vi "Variant to JSON Text (inline TEST).vi"(5 "enable LabVIEW extensions? (T)":bool=TRUE, 6 "Pretty Print?":bool, 8 "error in (no error)":errorcluster, 10 "Variant":variant) -> (0 "error out":errorcluster, 3 "<JSON>":string)   [LabVIEW 2013, in "JSONtext.lvlib"]
doc: "Converts a LabVIEW datatype (<b>Variant</b>) into a JSON value. Clusters are converted to JSON Objects, or to an Array if the first cluster element is unnamed."
uses:
  JSONtext.lvlib
  support/Infinity&NaN.ctl
  <vilib>/Utility/VariantDataType/RefnumType.ctl
  <vilib>/Utility/VariantDataType/VariantType.lvlib
  support/JSONtext support.lvlib
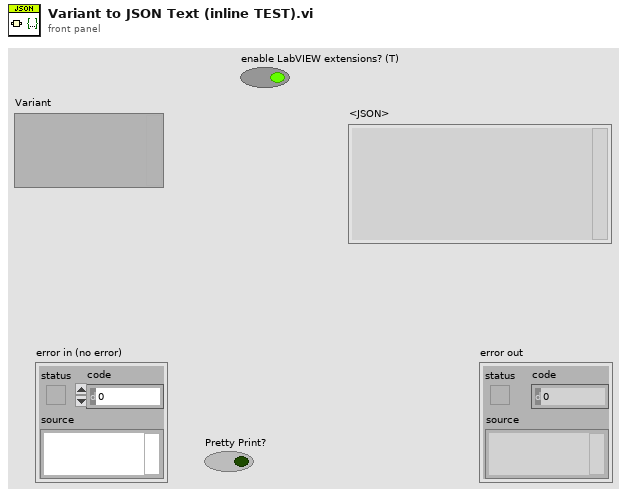
[diagram p1: front panel]
types:
  T1 = typedef "JSONtext support.lvlib/Infinity&NaN.ctl" = enum16{"Default (null)", "Extended", "LabVIEW extensions"}
  T2 = typedef "VariantType.lvlib/Type.ctl" = enum8{"Invalid Type", "Void", "I8", "I16", "I32", "I64", "U8", "U16", "U32", "U64", "Single Float", "Double Float", "Extended Float", "Single Complex", "Double Complex", "Extended Complex", "Enum U8", "Enum U16", "Enum U32", "Enum U64", "Single Float With Unit", "Double Float With Unit", "Extended Float With Unit", "Single Complex with Unit", "Double Complex with Unit", "Extended Complex with Unit", "Boolean", "String", "Path", "Picture", "Tag", "Array", "Cluster", "Variant", "LV Variant", "Waveform", "Timestamp", "Digital Waveform", "Digital Data", "ExpressData", "Refnum", "External Data", "VI", "Poly VI", "LabVIEW Class Instance", "Fixed Point"}
  T3 = cluster{"<JSON>attributes":string, "t0":timestamp, "dt":dbl, "Y":dbl[]}
  T4 = typedef "VariantType.lvlib/RefnumType.ctl" = enum16{"NotARefnum", "UnknownRefnum", "Generic", "Datalog", "ByteStream", "Device", "Occurence", "TCPNetConnection", "Auto", "Menu", "Imaq", "Hardware", "DataSocket", "Visa", "IVI", "UDPNetConnection", "Notifier", "Queue", "Irda", "EventReg", "DotNet", "UserEvent", "Callback", "UNUSED_EMPTY_POSITION", "BlueToothNetConnection", "LVObjApp", "LVObjVI", "LVObjUnknown", "GenericClass", "UserDefinedRefnumTag", "DataValue", "RT FIFO", "TDMS File"}
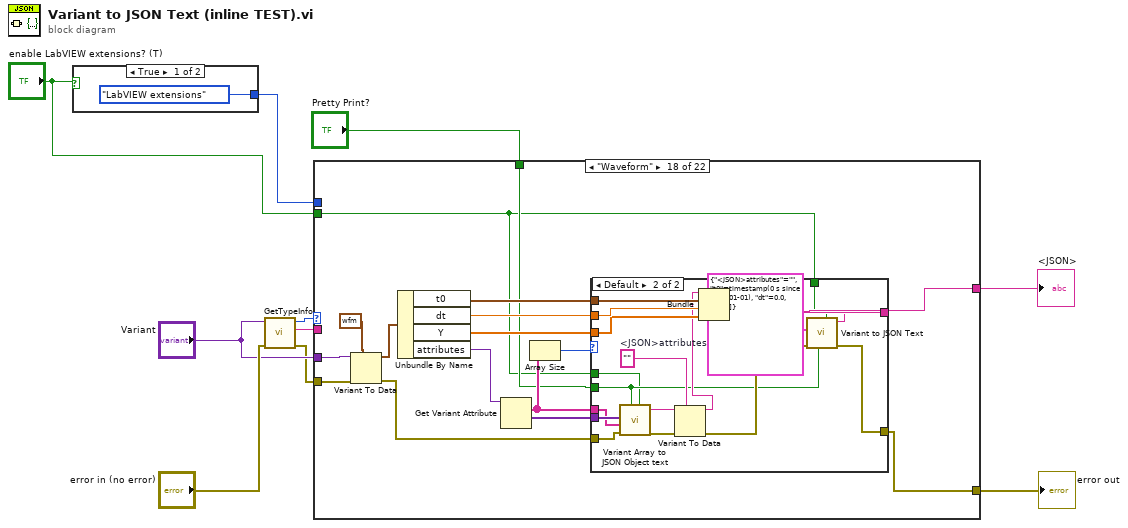
[diagram p0: block diagram]
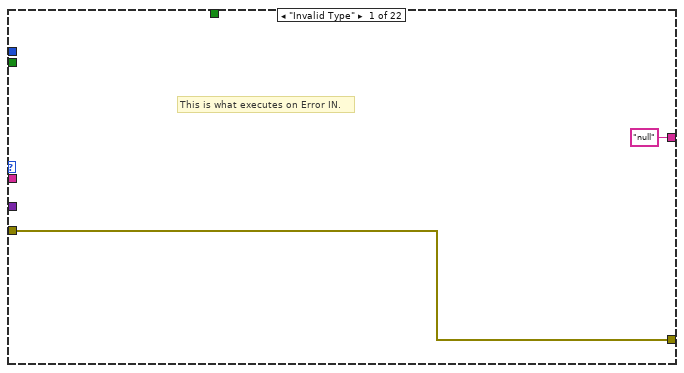
[diagram p2: hidden frame]
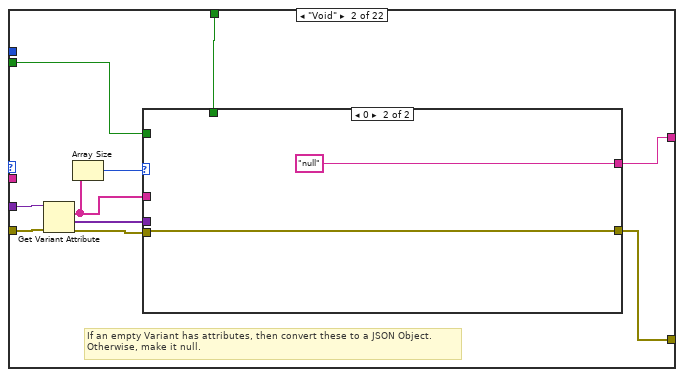
[diagram p3: hidden frame]
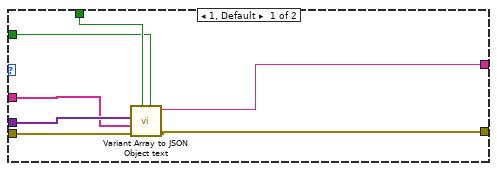
[diagram p4: hidden frame]
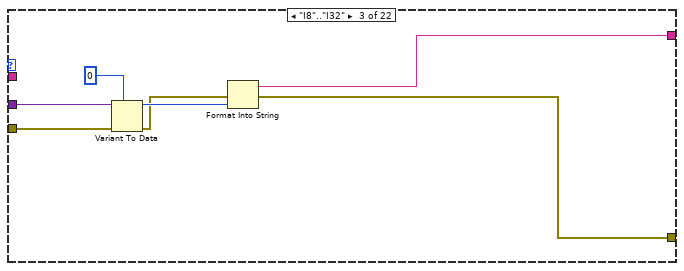
[diagram p5: hidden frame]
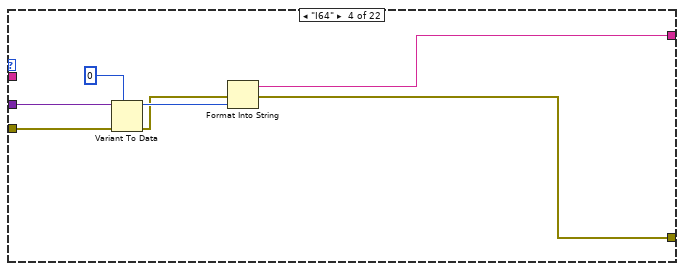
[diagram p6: hidden frame]
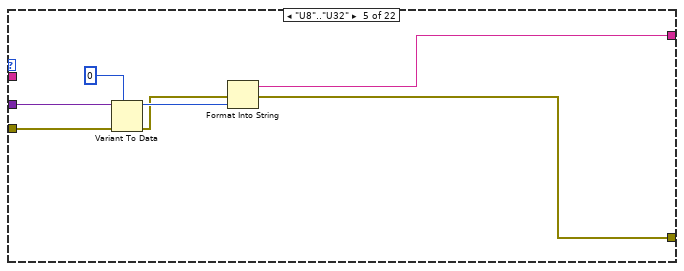
[diagram p7: hidden frame]
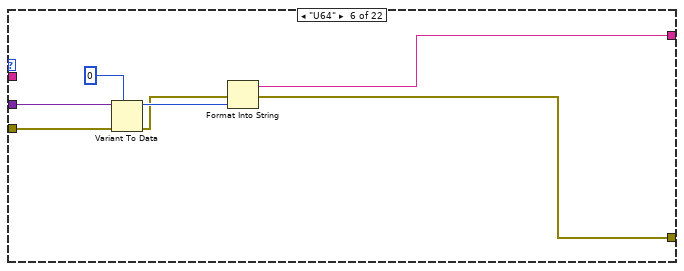
[diagram p8: hidden frame]
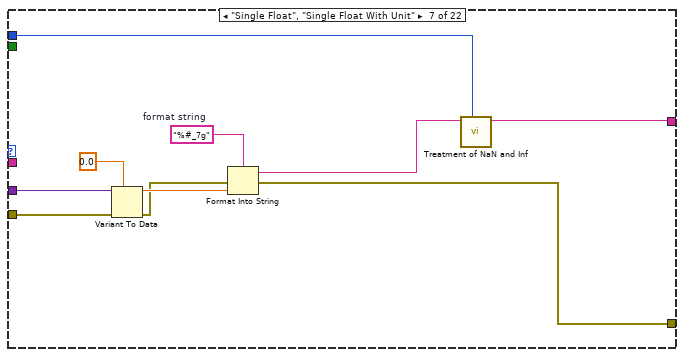
[diagram p9: hidden frame]
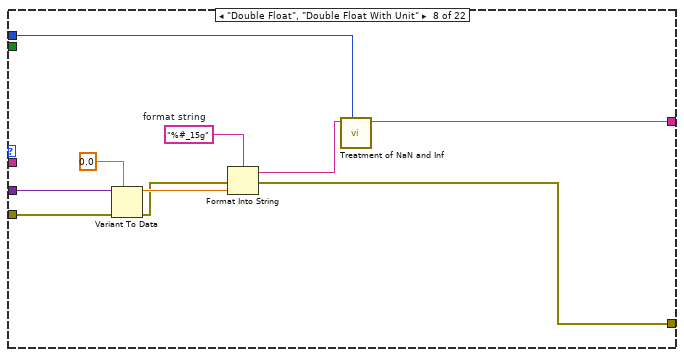
[diagram p10: hidden frame]
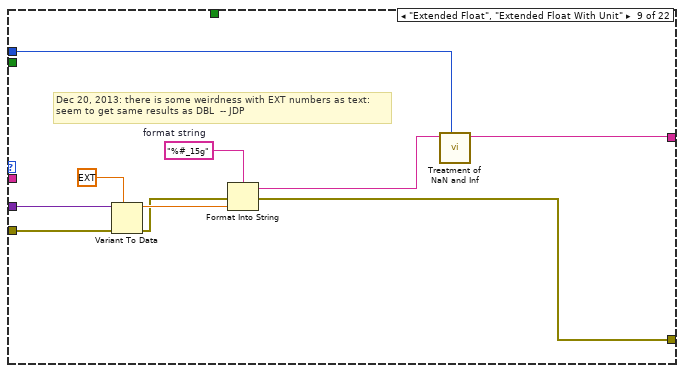
[diagram p11: hidden frame]
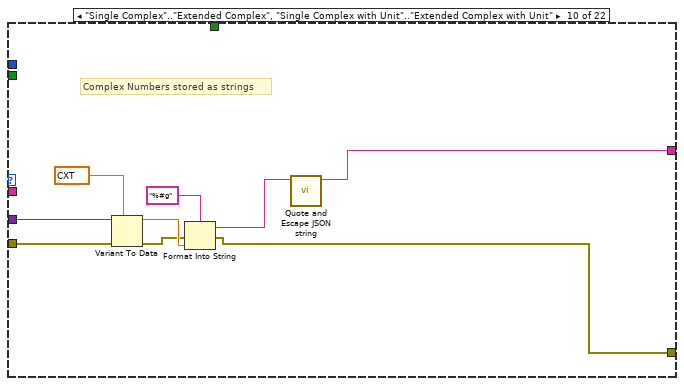
[diagram p12: hidden frame]
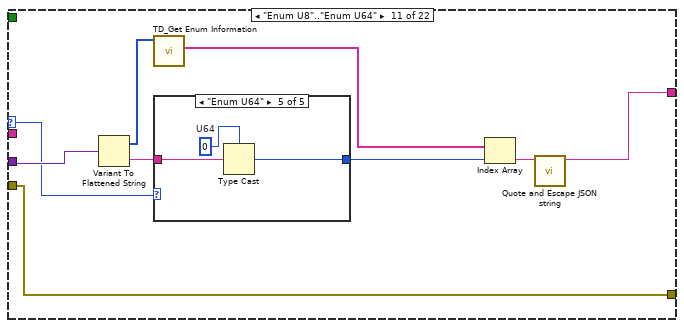
[diagram p13: hidden frame]
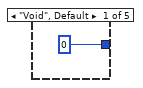
[diagram p14: hidden frame]
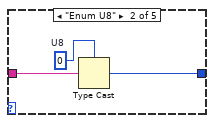
[diagram p15: hidden frame]
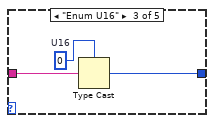
[diagram p16: hidden frame]
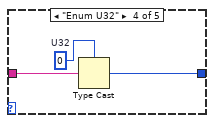
[diagram p17: hidden frame]
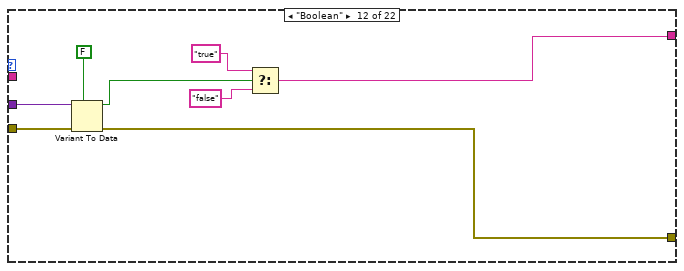
[diagram p18: hidden frame]
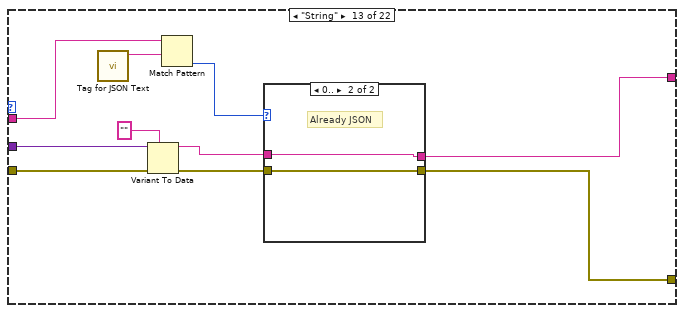
[diagram p19: hidden frame]
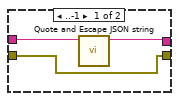
[diagram p20: hidden frame]
diagram:
  n1 = case shown="True" "enable LabVIEW extensions? (T)" {
    tunnel: [Infinity&NaN."LabVIEW extensions" ("Treatment of Infinity/NaN") Infinity&NaN."Default (null)" ("Treatment of Infinity/NaN")] -> w5
    frame True {
    }
    frame False {
    }
  }
  n2 = call <vilib>:"GetTypeInfo.vi"("error in (no error)"="error in (no error)", "Variant"="Variant") -> ("error out"=w3:errorcluster, "Name"=w1:string, "Type Enum"=w2:T2)  [unwired: 5 in, 2 out]
  n3 = case shown="\"Waveform\"" w2 {
    selector: w2 -> [_ _ _ _ _ _ _ _ _ _ w104 _ _ _ _ _ _ _ _ _ _ _]
    tunnel: "Variant" -> [_ w23 w40 w47 w54 w61 w71 w81 w91 w100 w105 w130 w140 w152 w163 w516 w533 w553 w588 w593 w619 w623]
    tunnel: [w13 w24 w34 w41 w48 w55 w66 w76 w86 w92 w101 w123 w136 w146 w164 w511 w537 w540 w580 w591 w612 w620] -> w9
    tunnel: w3 -> [w13 w18 w38 w45 w52 w59 w69 w79 w89 w99 w101 w128 w135 w150 w162 w514 w532 w552 w586 w592 w618 w620]
    tunnel: w1 -> [_ _ _ _ _ _ _ _ _ _ _ _ w133 _ w154 _ _ _ _ _ _ _]
    tunnel: w5 -> [_ _ _ _ _ _ w62 w72 w82 _ _ _ _ _ _ _ _ _ _ _ _ _]
    tunnel: ["null" ("<JSON>") w17 w36 w43 w50 w57 w63 w73 w83 w93 w102 w124 w131 w147 w156 w512 w529 w542 w581 w590 w615 w621] -> w7
    tunnel: "Pretty Print?" -> [_ w16 _ _ _ _ _ _ _ _ _ _ _ _ w157 w510 w531 w539 _ _ _ _]
    tunnel: "enable LabVIEW extensions? (T)" -> [_ w15 _ _ _ _ _ _ _ _ _ _ _ _ w155 w506 w530 w538 _ _ _ _]
    frame "Invalid Type" {
      # "This is what executes on Error IN."
    }
    frame "Void" {
      # "If an empty Variant has attributes, then convert these to a JSON Object.\nOtherwise, make it null."
      n4 = Get Variant Attribute(Variant=w23, error in=w18) -> (names=w21:string[], values=w20:variant[], error out=w19:errorcluster)  [unwired: 2 in, 1 out]
      n5 = Array Size(array=w21) -> (size(s)=w22:i32)
      n6 = case shown="0" w22 {
        tunnel: [w28 w32] -> w24
        tunnel: w21 -> [w30 _]
        tunnel: w20 -> [w31 _]
        tunnel: w19 -> [w29 w32]
        tunnel: [w27 "null"] -> w17
        tunnel: w16 -> [w26 _]
        tunnel: w15 -> [w25 _]
        frame 1, Default {
          n7 = call "Variant Array to JSON Object text.vi"("enable LabVIEW extensions? (T)"=w25, "Pretty Print?"=w26, "error in (no error)"=w29, "Names"=w30, "Array"=w31) -> ("error out"=w28:errorcluster, "<JSON>Object Text"=w27:string)  [unwired: 5 in]
        }
        frame 0 {
        }
      }
    }
    frame "I8".."I32" {
      n8 = Variant To Data(error in=w38, type=0, Variant=w40) -> (data=w37:i32, error out=w35:errorcluster)
      n9 = Format Into String(error in=w35, w37) -> (resulting string=w36:string, error out=w34:errorcluster)  [unwired: 2 in]
    }
    frame "I64" {
      n10 = Variant To Data(error in=w45, type=i64 0, Variant=w47) -> (data=w44:i64, error out=w42:errorcluster)
      n11 = Format Into String(error in=w42, w44) -> (resulting string=w43:string, error out=w41:errorcluster)  [unwired: 2 in]
    }
    frame "U8".."U32" {
      n12 = Variant To Data(error in=w52, type=u32 0, Variant=w54) -> (data=w51:u32, error out=w49:errorcluster)
      n13 = Format Into String(error in=w49, w51) -> (resulting string=w50:string, error out=w48:errorcluster)  [unwired: 2 in]
    }
    frame "U64" {
      n14 = Variant To Data(error in=w59, type=u64 0, Variant=w61) -> (data=w58:u64, error out=w56:errorcluster)
      n15 = Format Into String(error in=w56, w58) -> (resulting string=w57:string, error out=w55:errorcluster)  [unwired: 2 in]
    }
    frame "Single Float", "Single Float With Unit" {
      w65 = "%#_7g"  # format string
      n16 = Variant To Data(error in=w69, type=sgl 0.0, Variant=w71) -> (data=w68:sgl, error out=w67:errorcluster)
      n17 = Format Into String(format string=w65, error in=w67, w68) -> (resulting string=w64:string, error out=w66:errorcluster)  [unwired: 1 in]
      n18 = call "Treatment of NaN and Inf.vi"("Treatment of Infinity/NaN"=w62, "Numeric Text"=w64) -> ("<JSON>"=w63:string)  [unwired: 9 in]
    }
    frame "Double Float", "Double Float With Unit" {
      w75 = "%#_15g"  # format string
      n19 = Variant To Data(error in=w79, type=0.0, Variant=w81) -> (data=w78:dbl, error out=w77:errorcluster)
      n20 = Format Into String(format string=w75, error in=w77, w78) -> (resulting string=w74:string, error out=w76:errorcluster)  [unwired: 1 in]
      n21 = call "Treatment of NaN and Inf.vi"("Treatment of Infinity/NaN"=w72, "Numeric Text"=w74) -> ("<JSON>"=w73:string)  [unwired: 9 in]
    }
    frame "Extended Float", "Extended Float With Unit" {
      w85 = "%#_15g"  # format string
      # "Dec 20, 2013: there is some weirdness with EXT numbers as text:\nseem to get same results as DBL  -- JDP"
      n22 = Variant To Data(error in=w89, type=ext 0.0, Variant=w91) -> (data=w88:ext, error out=w87:errorcluster)
      n23 = Format Into String(format string=w85, error in=w87, w88) -> (resulting string=w84:string, error out=w86:errorcluster)  [unwired: 1 in]
      n24 = call "Treatment of NaN and Inf.vi"("Treatment of Infinity/NaN"=w82, "Numeric Text"=w84) -> ("<JSON>"=w83:string)  [unwired: 9 in]
    }
    frame "Single Complex".."Extended Complex", "Single Complex with Unit".."Extended Complex with Unit" {
      # "Complex Numbers stored as strings"
      n25 = Variant To Data(error in=w99, type=cxt 0.0+0.0i, Variant=w100) -> (data=w97:cxt, error out=w96:errorcluster)
      n26 = Format Into String(format string="%#g", error in=w96, w97) -> (resulting string=w94:string, error out=w92:errorcluster)  [unwired: 1 in]
      n27 = call "Quote and Escape JSON string.vi"("Plain Text"=w94) -> ("<JSON>"=w93:string)  [unwired: 10 in]
    }
    frame "Enum U8".."Enum U64" {
      n28 = Variant To Flattened String(Variant=w105) -> (data string=w108:string, 1:w109:i16[])
      n29 = call <vilib>:"TD_Get Enum Information.vi"("Type descriptor"=w109) -> ("Value Names"=w107:string[])  [unwired: 9 in, 1 out]
      n30 = case shown="\"Enum U64\"" w104 {
        tunnel: w108 -> [_ w113 w116 w119 w122]
        tunnel: [u64 0 ("U8") w111 w114 w117 w120] -> w106
        frame "Void", Default {
        }
        frame "Enum U8" {
          w112 = u8 0  # U8
          n31 = Type Cast(type=w112, x=w113) -> (*(type *) &x=w111:u8)
        }
        frame "Enum U16" {
          w115 = u16 0  # U16
          n32 = Type Cast(type=w115, x=w116) -> (*(type *) &x=w114:u16)
        }
        frame "Enum U32" {
          w118 = u32 0  # U32
          n33 = Type Cast(type=w118, x=w119) -> (*(type *) &x=w117:u32)
        }
        frame "Enum U64" {
          w121 = u64 0  # U64
          n34 = Type Cast(type=w121, x=w122) -> (*(type *) &x=w120:u64)
        }
      }
      n35 = Index Array(array=w107, index=w106) -> (element=w103:string)
      n36 = call "Quote and Escape JSON string.vi"("Plain Text"=w103) -> ("<JSON>"=w102:string)  [unwired: 10 in]
    }
    frame "Boolean" {
      n37 = Variant To Data(error in=w128, type=FALSE, Variant=w130) -> (data=w125:bool, error out=w123:errorcluster)
      n38 = Select(t="true", s=w125, f="false") -> (s? t:f=w124:string)
    }
    frame "String" {
      n39 = call "Tag for JSON Text.vi"() -> ("Tag for JSON text"=w134:string)  [unwired: 11 in]
      n40 = Variant To Data(error in=w135, type="", Variant=w140) -> (data=w138:string, error out=w137:errorcluster)
      n41 = Match Pattern(string=w133, regular expression=w134) -> (offset past match=w132:i32)  [unwired: 1 in, 3 out]
      n42 = case shown="0.." w132 {
        tunnel: w138 -> [w143 w144]
        tunnel: w137 -> [w141 w145]
        tunnel: [w141 w145] -> w136
        tunnel: [w142 w144] -> w131
        frame ..-1 {
          n43 = call "Quote and Escape JSON string.vi"("Plain Text"=w143) -> ("<JSON>"=w142:string)  [unwired: 10 in]
        }
        frame 0.. {
          # "Already JSON"
        }
      }
    }
    frame "Path" {
      n44 = Variant To Data(error in=w150, type=path "", Variant=w152) -> (data=w149:path, error out=w146:errorcluster)
      n45 = Path To String(path=w149) -> (string=w148:string)
      n46 = call "Quote and Escape JSON string.vi"("Plain Text"=w148) -> ("<JSON>"=w147:string)  [unwired: 10 in]
    }
    frame "Array" {
      n47 = call <vilib>:"GetArrayInfo.vi"("error in (no error)"=w162, "Variant"=w163) -> ("error out"=w160:errorcluster, "ArrayElement"=w159:variant, "NDims"=w161:i32)  [unwired: 6 in, 1 out]
      n48 = call <vilib>:"GetTypeInfo.vi"("error in (no error)"=w160, "Variant"=w159) -> ("error out"=w158:errorcluster, "Type Enum"=w153:T2)  [unwired: 5 in, 3 out]
      n49 = case shown="Default" w153 {
        tunnel: [w165 w175 w404] -> w164
        tunnel: w163 -> [_ w174 w403]
        tunnel: w161 -> [_ w173 w402]
        tunnel: w158 -> [w165 w172 w401]
        tunnel: w153 -> [_ w171 _]
        tunnel: w157 -> [_ w170 w400]
        tunnel: ["null" ("JSON Object Text out") w169 w399] -> w156
        tunnel: w155 -> [_ w168 w398]
        tunnel: w154 -> [_ w167 w396]
        frame "Invalid Type" {
        }
        frame Default {
          n50 = case shown="1" w173 {
            selector: w173 -> [_ _ _ _ _ w388]
            tunnel: [w182 w264 w347 w363 w379 w394] -> w175
            tunnel: w174 -> [w183 w265 w349 w365 w381 _]
            tunnel: w172 -> [w181 w263 w348 w364 w380 w393]
            tunnel: w171 -> [w180 w262 _ _ _ _]
            tunnel: w170 -> [w179 w261 w340 w356 w372 _]
            tunnel: [w178 w260 w346 w362 w378 "null" ("JSON Object Text out")] -> w169
            tunnel: w168 -> [w177 w259 w345 w361 w377 _]
            tunnel: w167 -> [w176 w258 _ _ _ _]
            frame 1 {
              n51 = case shown="Default" w180 {
                tunnel: w183 -> [w191 w212 w220 w227 w234 w241 w248 w257]
                tunnel: [w186 w207 w215 w222 w229 w236 w243 w250] -> w182
                tunnel: w181 -> [w189 w210 w218 w225 w232 w239 w246 w255]
                tunnel: w179 -> [_ _ _ _ _ _ _ w249]
                tunnel: [w185 w206 w214 w221 w228 w235 w242 w251] -> w178
                tunnel: w177 -> [w184 w205 _ _ _ _ _ w252]
                tunnel: w176 -> [_ _ _ _ _ _ _ _]
                frame "Single Float" {
                  n52 = Variant To Data(error in=w189, type=sgl[] [], Variant=w191) -> (data=w188:sgl[], error out=w187:errorcluster)
                  n53 = disable-structure shown="Enabled" {
                    disable-tunnel: w188 -> [w196 w199]
                    disable-tunnel: w187 -> [w195 w197]
                    disable-tunnel: [w194 w197] -> w186
                    disable-tunnel: [w193 w198] -> w185
                    disable-tunnel: w184 -> [w192 _]
                    frame Enabled {
                      # "Bug in 2015: Flatten to Json uses\nonly 18 significant figures for SGL\ndata (reported to NI)."
                      n54 = Flatten To JSON(enable LabVIEW extensions? (T)=w192, anything=w196, error in (no error)=w195) -> (JSON string=w193:string, 11:w194:errorcluster)
                    }
                    frame Disabled {
                      w204 = "%#_7g"  # format string
                      # "Not fast"
                      n55 = Array To Spreadsheet String(delimiter (Tab)=",", array=w199, 3:w204) -> (spreadsheet string=w202:string)
                      n56 = Concatenate Strings("[   " ("string"), w202, "]" ("string")) -> (w198:string)
                    }
                  }
                }
                frame "Double Float", "Extended Float" {
                  # "Bug in 2015: Flatten to Json uses\nonly 8 significant figures for EXT\ndata (reported to NI), so we \nconvert to DBLs"
                  n57 = Variant To Data(error in=w210, type=dbl[] [], Variant=w212) -> (data=w209:dbl[], error out=w208:errorcluster)
                  n58 = Flatten To JSON(enable LabVIEW extensions? (T)=w205, anything=w209, error in (no error)=w208) -> (JSON string=w206:string, 11:w207:errorcluster)
                }
                frame "Path" {
                  n59 = Variant To Data(error in=w218, type=path[] [], Variant=w220) -> (data=w217:path[], error out=w216:errorcluster)
                  n60 = Path To String(path=w217) -> (string=w213:string[])
                  n61 = Flatten To JSON(anything=w213, error in (no error)=w216) -> (JSON string=w214:string, 11:w215:errorcluster)  [unwired: 1 in]
                }
                frame "I8".."I32" {
                  n62 = Variant To Data(error in=w225, type=i32[] [], Variant=w227) -> (data=w224:i32[], error out=w223:errorcluster)
                  n63 = Flatten To JSON(anything=w224, error in (no error)=w223) -> (JSON string=w221:string, 11:w222:errorcluster)  [unwired: 1 in]
                }
                frame "I64" {
                  n64 = Variant To Data(error in=w232, type=i64[] [], Variant=w234) -> (data=w231:i64[], error out=w230:errorcluster)
                  n65 = Flatten To JSON(anything=w231, error in (no error)=w230) -> (JSON string=w228:string, 11:w229:errorcluster)  [unwired: 1 in]
                }
                frame "U8".."U32" {
                  n66 = Variant To Data(error in=w239, type=u32[] [], Variant=w241) -> (data=w238:u32[], error out=w237:errorcluster)
                  n67 = Flatten To JSON(anything=w238, error in (no error)=w237) -> (JSON string=w235:string, 11:w236:errorcluster)  [unwired: 1 in]
                }
                frame "U64" {
                  n68 = Variant To Data(error in=w246, type=u64[] [], Variant=w248) -> (data=w245:u64[], error out=w244:errorcluster)
                  n69 = Flatten To JSON(anything=w245, error in (no error)=w244) -> (JSON string=w242:string, 11:w243:errorcluster)  [unwired: 1 in]
                }
                frame Default {
                  n70 = Variant To Data(error in=w255, type=variant[] [], Variant=w257) -> (data=w253:variant[], error out=w254:errorcluster)
                  n71 = call "Variant Array to JSON Array text.vi"("enable LabVIEW extensions?"=w252, "Pretty Print?"=w249, "error in (no error)"=w254, "Array of Variants"=w253) -> ("error out"=w250:errorcluster, "<JSON>"=w251:string)  [unwired: 6 in]
                }
              }
            }
            frame 2 {
              n72 = case shown="Default" w262 {
                tunnel: w265 -> [w273 w294 w301 w308 w315 w322 w333]
                tunnel: [w268 w289 w296 w303 w310 w317 w325] -> w264
                tunnel: w263 -> [w271 w292 w299 w306 w313 w320 w331]
                tunnel: w261 -> [_ _ _ _ _ _ w323]
                tunnel: [w267 w288 w295 w302 w309 w316 w324] -> w260
                tunnel: w259 -> [w266 w287 _ _ _ _ w328]
                tunnel: w258 -> [_ _ _ _ _ _ _]
                frame "Single Float" {
                  n73 = Variant To Data(error in=w271, type=sgl[][] [], Variant=w273) -> (data=w270:sgl[][], error out=w269:errorcluster)
                  n74 = disable-structure shown="Enabled" {
                    disable-tunnel: w270 -> [w278 w281]
                    disable-tunnel: w269 -> [w277 w279]
                    disable-tunnel: [w276 w279] -> w268
                    disable-tunnel: [w275 w280] -> w267
                    disable-tunnel: w266 -> [w274 _]
                    frame Enabled {
                      # "Bug in 2015: Flatten to Json uses\nonly 18 significant figures for SGL\ndata (reported to NI)."
                      n75 = Flatten To JSON(enable LabVIEW extensions? (T)=w274, anything=w278, error in (no error)=w277) -> (JSON string=w275:string, 11:w276:errorcluster)
                    }
                    frame Disabled {
                      w286 = "%#_7g"  # format string
                      # "Not fast"
                      n76 = Array To Spreadsheet String(delimiter (Tab)=",", array=w281, 3:w286) -> (spreadsheet string=w284:string)
                      n77 = Concatenate Strings("[   " ("string"), w284, "]" ("string")) -> (w280:string)
                    }
                  }
                }
                frame "Double Float", "Extended Float" {
                  # "Bug in 2015: Flatten to Json uses\nonly 8 significant figures for EXT\ndata (reported to NI), so we \nconvert to DBLs"
                  n78 = Variant To Data(error in=w292, type=dbl[][] [], Variant=w294) -> (data=w291:dbl[][], error out=w290:errorcluster)
                  n79 = Flatten To JSON(enable LabVIEW extensions? (T)=w287, anything=w291, error in (no error)=w290) -> (JSON string=w288:string, 11:w289:errorcluster)
                }
                frame "I8".."I32" {
                  n80 = Variant To Data(error in=w299, type=i32[][] [], Variant=w301) -> (data=w298:i32[][], error out=w297:errorcluster)
                  n81 = Flatten To JSON(anything=w298, error in (no error)=w297) -> (JSON string=w295:string, 11:w296:errorcluster)  [unwired: 1 in]
                }
                frame "I64" {
                  n82 = Variant To Data(error in=w306, type=i64[][] [], Variant=w308) -> (data=w305:i64[][], error out=w304:errorcluster)
                  n83 = Flatten To JSON(anything=w305, error in (no error)=w304) -> (JSON string=w302:string, 11:w303:errorcluster)  [unwired: 1 in]
                }
                frame "U8".."U32" {
                  n84 = Variant To Data(error in=w313, type=u32[][] [], Variant=w315) -> (data=w312:u32[][], error out=w311:errorcluster)
                  n85 = Flatten To JSON(anything=w312, error in (no error)=w311) -> (JSON string=w309:string, 11:w310:errorcluster)  [unwired: 1 in]
                }
                frame "U64" {
                  n86 = Variant To Data(error in=w320, type=u64[][] [], Variant=w322) -> (data=w319:u64[][], error out=w318:errorcluster)
                  n87 = Flatten To JSON(anything=w319, error in (no error)=w318) -> (JSON string=w316:string, 11:w317:errorcluster)  [unwired: 1 in]
                }
                frame Default {
                  n88 = Variant To Data(error in=w331, type=variant[][] [], Variant=w333) -> (data=w326:variant[][], error out=w327:errorcluster)
                  n89 = for {
                    tunnel: w326 -> [w339] mode=indexing
                    tunnel: w323 -> [w338]
                    tunnel: [w334] -> w329 mode=indexing
                    shift-right: [w337] -> w330
                    shift-left: w327 -> [w336]
                    tunnel: w328 -> [w335]
                    n90 = call "Variant to JSON Text.vi"("enable LabVIEW extensions? (T)"=w335, "Pretty Print?"=w338, "error in (no error)"=w336, "Variant"=w339) -> ("error out"=w337:errorcluster, "<JSON>"=w334:string)  [unwired: 6 in]
                  }
                  n91 = call "Format JSON Array Text.vi"("Pretty Print?"=w323, "error in (no error)"=w330, "Array of JSON Text"=w329) -> ("error out"=w325:errorcluster, "<JSON>"=w324:string)  [unwired: 7 in]
                }
              }
            }
            frame 3 {
              n92 = Variant To Data(error in=w348, type=variant[][][] [], Variant=w349) -> (data=w343:variant[][][], error out=w342:errorcluster)
              n93 = for {
                tunnel: w343 -> [w355] mode=indexing
                shift-right: [w353] -> w347
                shift-left: w342 -> [w354]
                tunnel: [w350] -> w341 mode=indexing
                tunnel: w340 -> [w352]
                tunnel: w345 -> [w351]
                n94 = call "Variant to JSON Text.vi"("enable LabVIEW extensions? (T)"=w351, "Pretty Print?"=w352, "error in (no error)"=w354, "Variant"=w355) -> ("error out"=w353:errorcluster, "<JSON>"=w350:string)  [unwired: 6 in]
              }
              n95 = call "Format JSON Array Text.vi"("Pretty Print?"=w340, "Array of JSON Text"=w341) -> ("<JSON>"=w346:string)  [unwired: 8 in, 1 out]
            }
            frame 4 {
              n96 = Variant To Data(error in=w364, type=variant[][][][] [], Variant=w365) -> (data=w359:variant[][][][], error out=w358:errorcluster)
              n97 = for {
                tunnel: w359 -> [w371] mode=indexing
                shift-right: [w369] -> w363
                shift-left: w358 -> [w370]
                tunnel: [w366] -> w357 mode=indexing
                tunnel: w356 -> [w368]
                tunnel: w361 -> [w367]
                n98 = call "Variant to JSON Text.vi"("enable LabVIEW extensions? (T)"=w367, "Pretty Print?"=w368, "error in (no error)"=w370, "Variant"=w371) -> ("error out"=w369:errorcluster, "<JSON>"=w366:string)  [unwired: 6 in]
              }
              n99 = call "Format JSON Array Text.vi"("Pretty Print?"=w356, "Array of JSON Text"=w357) -> ("<JSON>"=w362:string)  [unwired: 8 in, 1 out]
            }
            frame 5 {
              n100 = Variant To Data(error in=w380, type=variant[][][][][] [], Variant=w381) -> (data=w375:variant[][][][][], error out=w374:errorcluster)
              n101 = for {
                tunnel: w375 -> [w387] mode=indexing
                shift-right: [w385] -> w379
                shift-left: w374 -> [w386]
                tunnel: [w382] -> w373 mode=indexing
                tunnel: w372 -> [w384]
                tunnel: w377 -> [w383]
                n102 = call "Variant to JSON Text.vi"("enable LabVIEW extensions? (T)"=w383, "Pretty Print?"=w384, "error in (no error)"=w386, "Variant"=w387) -> ("error out"=w385:errorcluster, "<JSON>"=w382:string)  [unwired: 6 in]
              }
              n103 = call "Format JSON Array Text.vi"("Pretty Print?"=w372, "Array of JSON Text"=w373) -> ("<JSON>"=w378:string)  [unwired: 8 in, 1 out]
            }
            frame Default {
              n104 = Format Into String(format string="Can't support array of dim=%d", w388) -> (resulting string=w391:string)  [unwired: 2 in, 1 out]
              n105 = call <vilib>:"Error Cluster From Error Code.vi"("error in (no error)"=w393, "error message (\"\")"=w391, "error code (0)"=1) -> ("error out"=w394:errorcluster)  [unwired: 6 in]
            }
          }
        }
        frame "String" {
          n106 = call "Tag for JSON Text.vi"() -> ("Tag for JSON text"=w397:string)  [unwired: 11 in]
          n107 = Match Pattern(string=w396, regular expression=w397) -> (offset past match=w395:i32)  [unwired: 1 in, 3 out]
          n108 = case shown="0.." w395 {
            tunnel: [w408 w477] -> w404
            tunnel: w403 -> [w411 w476]
            tunnel: w402 -> [w405 w475]
            tunnel: w401 -> [w410 w474]
            tunnel: w400 -> [w406 w473]
            tunnel: [w409 w472] -> w399
            tunnel: w398 -> [w407 w471]
            tunnel: w396 -> [_ w470]
            frame 0.. {
              # "Already JSON text, so\ncannot use Flatten to JSON primative"
              n109 = case shown="1" w405 {
                selector: w405 -> [w413 _ _ _]
                tunnel: w411 -> [_ w428 w445 w462]
                tunnel: w410 -> [w414 w427 w444 w461]
                tunnel: ["null" ("<JSON>") w420 w437 w454] -> w409
                tunnel: [w412 w421 w438 w455] -> w408
                tunnel: w407 -> [_ w422 w439 w456]
                tunnel: w406 -> [_ w419 w436 w453]
                frame 0, Default {
                  n110 = Format Into String(format string="Can't support array of dim=%d", w413) -> (resulting string=w416:string)  [unwired: 2 in, 1 out]
                  n111 = call <vilib>:"Error Cluster From Error Code.vi"("error in (no error)"=w414, "error message (\"\")"=w416, "error code (0)"=1) -> ("error out"=w412:errorcluster)  [unwired: 6 in]
                }
                frame 1 {
                  n112 = Variant To Data(error in=w427, type=variant[] [], Variant=w428) -> (data=w424:variant[], error out=w423:errorcluster)
                  n113 = for {
                    tunnel: w424 -> [w435] mode=indexing
                    tunnel: w419 -> [w434]
                    tunnel: [w430] -> w425 mode=indexing
                    shift-right: [w433] -> w426
                    shift-left: w423 -> [w432]
                    tunnel: w422 -> [w431]
                    n114 = call "Variant to JSON Text.vi"("enable LabVIEW extensions? (T)"=w431, "Pretty Print?"=w434, "error in (no error)"=w432, "Variant"=w435) -> ("error out"=w433:errorcluster, "<JSON>"=w430:string)  [unwired: 6 in]
                  }
                  n115 = call "Format JSON Array Text.vi"("Pretty Print?"=w419, "error in (no error)"=w426, "Array of JSON Text"=w425) -> ("error out"=w421:errorcluster, "<JSON>"=w420:string)  [unwired: 7 in]
                }
                frame 2 {
                  n116 = Variant To Data(error in=w444, type=variant[][] [], Variant=w445) -> (data=w441:variant[][], error out=w440:errorcluster)
                  n117 = for {
                    tunnel: w441 -> [w452] mode=indexing
                    tunnel: w436 -> [w451]
                    tunnel: [w447] -> w442 mode=indexing
                    shift-right: [w450] -> w443
                    shift-left: w440 -> [w449]
                    tunnel: w439 -> [w448]
                    n118 = call "Variant to JSON Text.vi"("enable LabVIEW extensions? (T)"=w448, "Pretty Print?"=w451, "error in (no error)"=w449, "Variant"=w452) -> ("error out"=w450:errorcluster, "<JSON>"=w447:string)  [unwired: 6 in]
                  }
                  n119 = call "Format JSON Array Text.vi"("Pretty Print?"=w436, "error in (no error)"=w443, "Array of JSON Text"=w442) -> ("error out"=w438:errorcluster, "<JSON>"=w437:string)  [unwired: 7 in]
                }
                frame 3 {
                  n120 = Variant To Data(error in=w461, type=variant[][][] [], Variant=w462) -> (data=w458:variant[][][], error out=w457:errorcluster)
                  n121 = for {
                    tunnel: w458 -> [w469] mode=indexing
                    tunnel: w453 -> [w468]
                    tunnel: [w464] -> w459 mode=indexing
                    shift-right: [w467] -> w460
                    shift-left: w457 -> [w466]
                    tunnel: w456 -> [w465]
                    n122 = call "Variant to JSON Text.vi"("enable LabVIEW extensions? (T)"=w465, "Pretty Print?"=w468, "error in (no error)"=w466, "Variant"=w469) -> ("error out"=w467:errorcluster, "<JSON>"=w464:string)  [unwired: 6 in]
                  }
                  n123 = call "Format JSON Array Text.vi"("Pretty Print?"=w453, "error in (no error)"=w460, "Array of JSON Text"=w459) -> ("error out"=w455:errorcluster, "<JSON>"=w454:string)  [unwired: 7 in]
                }
              }
            }
            frame ..-1 {
              n124 = case shown="1" w475 {
                selector: w475 -> [_ _ _ w499]
                tunnel: [w483 w490 w497 w505] -> w477
                tunnel: w476 -> [w484 w491 w498 _]
                tunnel: w474 -> [w482 w489 w496 w504]
                tunnel: w473 -> [_ _ _ _]
                tunnel: [w481 w488 w495 "null" ("JSON Object Text out")] -> w472
                tunnel: w471 -> [_ _ _ _]
                tunnel: w470 -> [_ _ _ _]
                frame 1 {
                  n125 = Variant To Data(error in=w482, type=string[] [], Variant=w484) -> (data=w479:string[], error out=w478:errorcluster)
                  n126 = Flatten To JSON(anything=w479, error in (no error)=w478) -> (JSON string=w481:string, 11:w483:errorcluster)  [unwired: 1 in]
                }
                frame 2 {
                  n127 = Variant To Data(error in=w489, type=string[][] [], Variant=w491) -> (data=w486:string[][], error out=w485:errorcluster)
                  n128 = Flatten To JSON(anything=w486, error in (no error)=w485) -> (JSON string=w488:string, 11:w490:errorcluster)  [unwired: 1 in]
                }
                frame 3 {
                  n129 = Variant To Data(error in=w496, type=string[][][] [], Variant=w498) -> (data=w493:string[][][], error out=w492:errorcluster)
                  n130 = Flatten To JSON(anything=w493, error in (no error)=w492) -> (JSON string=w495:string, 11:w497:errorcluster)  [unwired: 1 in]
                }
                frame Default {
                  n131 = Format Into String(format string="Can't support array of dim=%d", w499) -> (resulting string=w502:string)  [unwired: 2 in, 1 out]
                  n132 = call <vilib>:"Error Cluster From Error Code.vi"("error in (no error)"=w504, "error message (\"\")"=w502, "error code (0)"=1) -> ("error out"=w505:errorcluster)  [unwired: 6 in]
                }
              }
            }
          }
        }
      }
    }
    frame "Cluster" {
      # "Cluster of unnamed (possibly with <JSON>tags) to JSON Array?"
      n133 = Variant To Data(error in=w514, type=variant[] [], Variant=w516) -> (data=w509:variant[], error out=w515:errorcluster)
      n134 = Index Array(array=w509) -> (element=w508:variant)  [unwired: 1 in]
      n135 = call <vilib>:"GetTypeInfo.vi"("Variant"=w508) -> ("Name"=w507:string)  [unwired: 6 in, 4 out]
      n136 = case shown="Default" w507 {
        tunnel: w515 -> [w522 w525]
        tunnel: [w521 w528] -> w512
        tunnel: [w520 w526] -> w511
        tunnel: w510 -> [w519 w523]
        tunnel: w509 -> [w518 w524]
        tunnel: w506 -> [w517 w527]
        frame Default {
          n137 = call "Variant Array to JSON Object text.vi"("enable LabVIEW extensions? (T)"=w517, "Pretty Print?"=w519, "error in (no error)"=w522, "Array"=w518) -> ("error out"=w520:errorcluster, "<JSON>Object Text"=w521:string)  [unwired: 6 in]
        }
        frame "", "<JSON>" {
          n138 = call "Variant Array to JSON Array text.vi"("enable LabVIEW extensions?"=w527, "Pretty Print?"=w523, "error in (no error)"=w525, "Array of Variants"=w524) -> ("error out"=w526:errorcluster, "<JSON>"=w528:string)  [unwired: 6 in]
        }
      }
    }
    frame "Variant", "LV Variant" {
      n139 = Variant To Data(error in=w532, type=variant, Variant=w533) -> (data=w536:variant, error out=w535:errorcluster)
      n140 = call "Variant to JSON Text.vi"("enable LabVIEW extensions? (T)"=w530, "Pretty Print?"=w531, "error in (no error)"=w535, "Variant"=w536) -> ("error out"=w537:errorcluster, "<JSON>"=w529:string)  [unwired: 6 in]
    }
    frame "Waveform" {
      n141 = Variant To Data(error in=w552, type=waveform(dbl) {"t0"=timestamp(0 s since 1904-01-01), "dt"=1.0, "Y"=[]} ("waveform"), Variant=w553) -> (data=w550:waveform(dbl), error out=w541:errorcluster)
      n142 = Unbundle By Name(w550) -> ("t0"=w549:timestamp, "dt"=w548:dbl, "Y"=w547:dbl[], "attributes"=w546:variant)
      n143 = Get Variant Attribute(Variant=w546) -> (names=w543:string[], values=w544:variant[])  [unwired: 3 in, 2 out]
      n144 = Array Size(array=w543) -> (size(s)=w545:i32)
      n145 = case shown="Default" w545 {
        tunnel: w549 -> [w562 w579]
        tunnel: w548 -> [w561 w578]
        tunnel: w547 -> [w560 w577]
        tunnel: [w554 w563] -> w542
        tunnel: w544 -> [_ w576]
        tunnel: w543 -> [_ w575]
        tunnel: w539 -> [w555 w565]
        tunnel: w541 -> [w558 w568]
        tunnel: [w557 w571] -> w540
        tunnel: w538 -> [w556 w566]
        tunnel: w538 -> [_ w564]
        frame 0 {
          n146 = Bundle("t0"=w562, "dt"=w561, "Y"=w560) -> (w559:cluster{"t0":timestamp, "dt":dbl, "Y":dbl[]})  [unwired: 1 in]
          n147 = call "Variant to JSON Text.vi"("enable LabVIEW extensions? (T)"=w556, "Pretty Print?"=w555, "error in (no error)"=w558, "Variant"=w559) -> ("error out"=w557:errorcluster, "<JSON>"=w554:string)  [unwired: 6 in]
        }
        frame Default {
          (unwired) T3 {"<JSON>attributes"="", "t0"=timestamp(0 s since 1904-01-01), "dt"=0.0, "Y"=[]} ("output cluster")
          w573 = ""  # <JSON>attributes
          n148 = call "Variant Array to JSON Object text.vi"("enable LabVIEW extensions? (T)"=w564, "Pretty Print?"=w565, "error in (no error)"=w568, "Names"=w575, "Array"=w576) -> ("error out"=w569:errorcluster, "<JSON>Object Text"=w574:string)  [unwired: 5 in]
          n149 = Variant To Data(error in=w569, type=w573, Variant=w574) -> (data=w567:string, error out=w570:errorcluster)
          n150 = Bundle("<JSON>attributes"=w567, "t0"=w579, "dt"=w578, "Y"=w577) -> (w572:T3)  [unwired: 1 in]
          n151 = call "Variant to JSON Text.vi"("enable LabVIEW extensions? (T)"=w566, "Pretty Print?"=w565, "error in (no error)"=w570, "Variant"=w572) -> ("error out"=w571:errorcluster, "<JSON>"=w563:string)  [unwired: 6 in]
        }
      }
    }
    frame "Timestamp" {
      n152 = Variant To Data(error in=w586, type=timestamp(0 s since 1904-01-01), Variant=w588) -> (data=w583:timestamp, error out=w580:errorcluster)
      n153 = Format Date/Time String(time format string (%c)="%Y-%m-%dT%H:%M:%S%3uZ", seconds (now)=w583, UTC format=TRUE) -> (date/time string=w582:string)
      n154 = call "Quote and Escape JSON string.vi"("Plain Text"=w582) -> ("<JSON>"=w581:string)  [unwired: 10 in]
    }
    frame "Refnum" {
      (unwired) RefnumType."NotARefnum" ("ReferenceType")
      n155 = call <vilib>:"GetRefnumInfo.vi"("error in (no error)"=w592, "Variant"=w593) -> ("error out"=w595:errorcluster, "ReferenceType"=w594:T4)  [unwired: 6 in, 2 out]
      n156 = case shown="Default" w594 {
        selector: w594 -> [_ _ w606]
        tunnel: ["null" w599 w607] -> w589
        tunnel: w595 -> [w596 w601 w609]
        tunnel: [w596 w598 w608] -> w591
        tunnel: w593 -> [_ w602 w611]
        frame "NotARefnum", "UnknownRefnum" {
        }
        frame "Visa", "IVI", "UserDefinedRefnumTag" {
          n157 = Variant To Data(error in=w601, type="", Variant=w602) -> (data=w599:string, error out=w598:errorcluster)
        }
        frame Default {
          # "Store refnums in Hex (use case: routing back replies)"
          n158 = Variant To Flattened String(Variant=w611) -> (data string=w610:string)  [unwired: 1 out]
          n159 = Type Cast(type=u32 0, x=w610) -> (*(type *) &x=w603:u32)
          n160 = Format Into String(format string="%s->%x", error in=w609, w606, w603) -> (resulting string=w607:string, error out=w608:errorcluster)  [unwired: 1 in]
        }
      }
      n161 = call "Quote and Escape JSON string.vi"("Plain Text"=w589) -> ("<JSON>"=w590:string)  [unwired: 10 in]
    }
    frame "LabVIEW Class Instance" {
      # "Classes saved in flattened form as strings"
      n162 = Variant To Data(error in=w618, type=refnum<class> refnum ("LabVIEW Object"), Variant=w619) -> (data=w616:refnum<class>, error out=w613:errorcluster)
      n163 = Flatten To String(anything=w616, error in (no error)=w613) -> (data string=w614:string, error out=w612:errorcluster)  [unwired: 2 in, 1 out]
      n164 = call "Quote and Escape JSON string.vi"("Plain Text"=w614) -> ("<JSON>"=w615:string)  [unwired: 10 in]
    }
    frame Default {
      # "For lack of a better thing to do,\nflatten to string."
      n165 = Variant To Flattened String(Variant=w623) -> (data string=w622:string)  [unwired: 1 out]
      n166 = call "Quote and Escape JSON string.vi"("Plain Text"=w622) -> ("<JSON>"=w621:string)  [unwired: 10 in]
    }
  }
  "error out" <- w9
  "<JSON>" <- w7
